vi "p1.vi"() -> ()   [LabVIEW 2023, in "d4.lvlib"]
uses:
  d4.lvlib
  dc8a3cb4-4444-413c-ac1b-c32ca85782e5.vi
  <vilib>/regexp/Match Regular Expression.xnode
  AOC/AOC.lvlib
panel:
  in  "Example":string="Card 1: 41 48 83 86 17 | 83 86  6 31 17  9 48 53\nCard 2: 13 32 20 16 61 | 61 30 68 82 17 32 24 19\nCard 3:  1 21 53 59 44 | 69 82 63 72 16 21 14  1\nCard 4: 41 92 73 84 69 | 59 84 76 51 58  5 54 83\nCard 5: 87 83 26 28 32 | 88 30 70 12 93 22 82 36\nCard 6: 31 18 13 56 72 | 74 77 10 23 35 67 36 11"
  in  "Example":bool
  out "Answer":i64=605
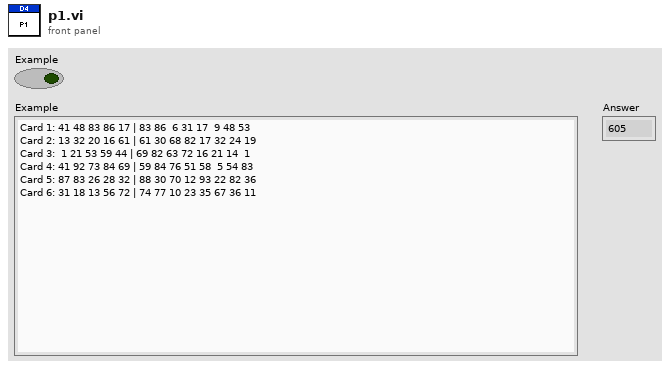
[diagram p1: front panel]
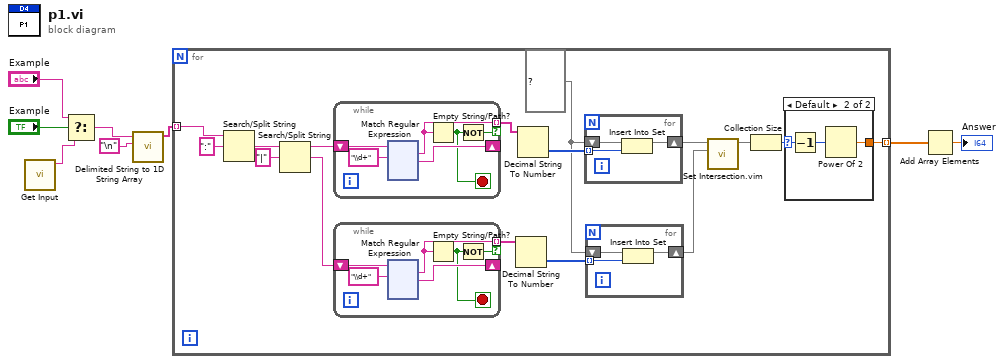
[diagram p0: block diagram]
diagram:
  n1 = call "Get Input.vi"() -> ("Input"=w8:string)  [unwired: 11 in]
  n2 = Select(t="Example", s="Example", f=w8) -> (s? t:f=w7:string)
  n3 = call <vilib>:"Delimited String to 1D String Array.vi"("delimiter"="\n", "delimited string"=w7) -> ("string array"=w2:string[])  [unwired: 9 in]
  n4 = for {
    tunnel: w2 -> [w24] mode=indexing
    tunnel: [w11] -> w1 mode=indexing
    w17 = set{i32} {} ("set")
    n5 = Search/Split String(string=w24, search string/char (-)=":") -> (match + rest of string=w22:string)  [unwired: 1 in, 2 out]
    n6 = Search/Split String(string=w22, search string/char (-)="|") -> (substring before match=w20:string, match + rest of string=w10:string)  [unwired: 1 in, 1 out]
    n7 = while {
      shift-right: [w151] -> _
      shift-left: w20 -> [w153]
      tunnel: [w150] -> w19 mode=indexing if=w148
      stop <- w149 stop-if-true
      n8 = xnode "Match Regular Expression"("input string"=w153, "regular expression"="\\d+") -> ("whole match"=w150:string, "after match"=w151:string)  [unwired: 4 in, 3 out]
      n9 = Empty String/Path?(string/path=w150) -> (empty?=w149:bool)
      n10 = Not(x=w149) -> (.not. x?=w148:bool)
    }
    n11 = while {
      shift-right: [w28] -> _
      shift-left: w10 -> [w30]
      tunnel: [w27] -> w9 mode=indexing if=w25
      stop <- w26 stop-if-true
      n12 = xnode "Match Regular Expression"("input string"=w30, "regular expression"="\\d+") -> ("whole match"=w27:string, "after match"=w28:string)  [unwired: 4 in, 3 out]
      n13 = Empty String/Path?(string/path=w27) -> (empty?=w26:bool)
      n14 = Not(x=w26) -> (.not. x?=w25:bool)
    }
    n15 = Decimal String To Number(string=w9) -> (number=w16:i32[])  [unwired: 2 in, 1 out]
    n16 = Decimal String To Number(string=w19) -> (number=w18:i32[])  [unwired: 2 in, 1 out]
    n17 = for {
      tunnel: w18 -> [w278] mode=indexing
      shift-right: [w279] -> w15
      shift-left: w17 -> [w280]
      n18 = Insert Into Set(10:w278, 11:w280) -> (3:w279:set{i32})  [unwired: 1 out]
    }
    n19 = for {
      tunnel: w16 -> [w275] mode=indexing
      shift-right: [w276] -> w14
      shift-left: w17 -> [w277]
      n20 = Insert Into Set(10:w275, 11:w277) -> (3:w276:set{i32})  [unwired: 1 out]
    }
    n21 = call "Set Intersection.vim"("set 2"=w14, "set 1"=w15) -> ("intersection"=w13:set{i32})  [unwired: 9 in]
    n22 = Collection Size(1:w13) -> (0:w12:i32)
    n23 = case shown="Default" w12 {
      selector: w12 -> [w271 w274]
      tunnel: [w271 w272] -> w11
      frame 0 {
      }
      frame Default {
        n24 = Decrement(x=w274) -> (x-1=w273:i32)
        n25 = Power Of 2(x=w273) -> (2^x=w272:dbl)
      }
    }
  }
  n26 = Add Array Elements(numeric array=w1) -> (sum=→"Answer":dbl)
